vi "Nanonis_SR830_ExternalDevice.vi"(1 "Output Amp #1":dbl=1.0, 2 "Output Amp #2":dbl=1.0, 3 "Output Amp #3":dbl=1.0) -> (7 "X-Value":dbl, 8 "X-Value 2":dbl, 9 "Theta-Value":dbl, 10 "Theta-Value 2":dbl)   [LabVIEW 2021]
uses:
  <instrlib>/Stanford Research 830/Public/Data/Read (All Parameters).vi
  <instrlib>/Stanford Research 830/Stanford Research 830.lvlib
panel:
  in  "External Reference Trigger (0: Sine Zero Crossing)  2":u16(ring) items=["Sine Zero Crossing", "TTL Rising Edge", "TTL Falling Edge"]
  in  "External Reference Trigger (0: Sine Zero Crossing)":u16(ring) items=["Sine Zero Crossing", "TTL Rising Edge", "TTL Falling Edge"]
  in  "External Reference Trigger #2 (0: Sine Zero Crossing)":u16(ring) items=["Sine Zero Crossing", "TTL Rising Edge", "TTL Falling Edge"]
  out "SR830 #3 Sensitivity 3":dbl
  out "SR830 #3 Sensitivity 2":dbl
  out "SR830 #3 Sensitivity":dbl
  out "Sense\nOver 3":bool
  out "Sense\nUnder 3":bool
  out "Sense\nOver 2":bool
  out "Sense\nUnder 2":bool
  out "Sense Under":bool
  out "Sense Over":bool
  in  "Loop Timing (ms)":u32=500
  out "Reference Freq 3":dbl
  out "Theta-Value 3":dbl
  out "R-Value 3":dbl
  out "X-Value 3":dbl
  out "Reference Freq 2":dbl
  out "R-Value 2":dbl
  out "Reference Freq":dbl
  out "R-Value":dbl
  out "Device Intialization":T1
  in  "System #3 Enabled/Disabled":bool
  in  "SR830 #3":refnum<visa-resource-name>="GPIB0::10::INSTR"
  in  "SR830 #3 Input Connection":u16(ring) items=["Single-Ended Voltage", "Differential Voltage", "1 MOhm Current Gain", "100 MOhm Current Gain"]
  in  "SR830 #3\nInput Coupling":u16(ring) items=["AC", "DC"]
  in  "SR830 #3 Input \nShield Grounding":u16(ring) items=["Float", "Ground"]
  in  "SR830 #3 Input\nNotch Filter":u16(ring) items=["None", "Line Notch", "2x Line Notch", "Both Notch Filters"]
  in  "SR830 #3 Trigger Source":u16(ring) items=["Internal", "External"]
  in  "SR830 #3 Internal \nReference Frequency":dbl=17.0
  in  "SR830 #3 Detection Harm. Num.":dbl=1.0
  in  "SR830 #3 Reference Source":u16(ring) items=["External", "Internal"]
  in  "SR830 #3 Manual \nPhase":dbl
  in  "SR830 #3 \nAuto Phase":bool
  in  "SR830 #3 \nTime Constant":u16(ring)=9 items=["10 us", "30 us", "100 us", "300 us", "1 ms", "3 ms", "10 ms", "30 ms", "100 ms", "300 ms", "1 s", "3 s", "10 s", "30 s", "100 s", "300 s", "1 ks", "3 ks", "10 ks", "30 ks"]
  in  "SR830 #3 Low\nPass Filter Slope":u16(ring)=3 items=["6 dB/oct", "12 dB/oct", "18 db/oct", "24 dB/oct"]
  in  "SR830 #3\nSync Filter":bool
  in  "SR830 #3 \nDynamic Reserve":i16(ring)=1 items=["Auto Reserve"=-1, "High Reserve"=0, "Normal"=1, "Low Noise"=2]
  in  "SR830 #3 Initial\nSensitivity":i16(ring)=17 items=["Auto Gain"=-1, "2 nV/fA"=0, "5 nV/fA"=1, "10 nV/fA"=2, "20 nV/fA"=3, "50 nV/fA"=4, "100 nV/fA"=5, "200 nV/fA"=6, "500 nV/fA"=7, "1 uV/pA"=8, "2 uV/pA"=9, "5 uV/pA"=10, "10 uV/pA"=11, "20 uV/pA"=12, "50 uV/pA"=13, "100 uV/pA"=14, "200 uV/pA"=15, "500 uV/pA"=16, "1 mV/nA"=17, "2 mV/nA"=18, "5 mV/nA"=19, "10 mV/nA"=20, "20 mV/nA"=21, "50 mV/nA"=22, "100 mV/nA"=23, "200 mV/nA"=24, "500 mV/mA"=25, "1 V/uA"=26]
  in  "System #2 Enabled/Disabled":bool
  in  "SR830 #2":refnum<visa-resource-name>="GPIB0::10::INSTR"
  in  "SR830 #2 Input Connection":u16(ring)=1 items=["Single-Ended Voltage", "Differential Voltage", "1 MOhm Current Gain", "100 MOhm Current Gain"]
  in  "SR830 #2\nInput Coupling":u16(ring) items=["AC", "DC"]
  in  "SR830 #2 Input \nShield Grounding":u16(ring) items=["Float", "Ground"]
  in  "SR830 #2 Input\nNotch Filter":u16(ring) items=["None", "Line Notch", "2x Line Notch", "Both Notch Filters"]
  in  "SR830 #2 Trigger Source":u16(ring) items=["Internal", "External"]
  in  "SR830 #2 Internal \nReference Frequency":dbl=17.0
  in  "SR830 #2 Detection Harm. Num.":dbl=1.0
  in  "SR830 #2 Reference Source":u16(ring) items=["External", "Internal"]
  in  "SR830 #2 Manual \nPhase":dbl
  in  "SR830 #2 \nAuto Phase":bool
  in  "SR830 #2 \nTime Constant":u16(ring)=8 items=["10 us", "30 us", "100 us", "300 us", "1 ms", "3 ms", "10 ms", "30 ms", "100 ms", "300 ms", "1 s", "3 s", "10 s", "30 s", "100 s", "300 s", "1 ks", "3 ks", "10 ks", "30 ks"]
  in  "SR830 #2 Low\nPass Filter Slope":u16(ring)=3 items=["6 dB/oct", "12 dB/oct", "18 db/oct", "24 dB/oct"]
  in  "SR830 #2\nSync Filter":bool
  in  "SR830 #2 \nDynamic Reserve":i16(ring)=1 items=["Auto Reserve"=-1, "High Reserve"=0, "Normal"=1, "Low Noise"=2]
  in  "SR830 #2 Initial \nSensitivity":i16(ring)=17 items=["Auto Gain"=-1, "2 nV/fA"=0, "5 nV/fA"=1, "10 nV/fA"=2, "20 nV/fA"=3, "50 nV/fA"=4, "100 nV/fA"=5, "200 nV/fA"=6, "500 nV/fA"=7, "1 uV/pA"=8, "2 uV/pA"=9, "5 uV/pA"=10, "10 uV/pA"=11, "20 uV/pA"=12, "50 uV/pA"=13, "100 uV/pA"=14, "200 uV/pA"=15, "500 uV/pA"=16, "1 mV/nA"=17, "2 mV/nA"=18, "5 mV/nA"=19, "10 mV/nA"=20, "20 mV/nA"=21, "50 mV/nA"=22, "100 mV/nA"=23, "200 mV/nA"=24, "500 mV/mA"=25, "1 V/uA"=26]
  in  "SR830 #1 Initial\nSensitivity":i16(ring)=17 items=["Auto Gain"=-1, "2 nV/fA"=0, "5 nV/fA"=1, "10 nV/fA"=2, "20 nV/fA"=3, "50 nV/fA"=4, "100 nV/fA"=5, "200 nV/fA"=6, "500 nV/fA"=7, "1 uV/pA"=8, "2 uV/pA"=9, "5 uV/pA"=10, "10 uV/pA"=11, "20 uV/pA"=12, "50 uV/pA"=13, "100 uV/pA"=14, "200 uV/pA"=15, "500 uV/pA"=16, "1 mV/nA"=17, "2 mV/nA"=18, "5 mV/nA"=19, "10 mV/nA"=20, "20 mV/nA"=21, "50 mV/nA"=22, "100 mV/nA"=23, "200 mV/nA"=24, "500 mV/mA"=25, "1 V/uA"=26]
  in  "SR830 #1 \nDynamic Reserve":i16(ring)=1 items=["Auto Reserve"=-1, "High Reserve"=0, "Normal"=1, "Low Noise"=2]
  in  "SR830 #1\nSync Filter":bool
  in  "SR830 #1 Low\nPass Filter Slope":u16(ring)=3 items=["6 dB/oct", "12 dB/oct", "18 db/oct", "24 dB/oct"]
  in  "SR830 #1 \nTime Constant":u16(ring)=8 items=["10 us", "30 us", "100 us", "300 us", "1 ms", "3 ms", "10 ms", "30 ms", "100 ms", "300 ms", "1 s", "3 s", "10 s", "30 s", "100 s", "300 s", "1 ks", "3 ks", "10 ks", "30 ks"]
  in  "SR830 #1 \nAuto Phase":bool
  in  "SR830 #1 Manual \nPhase":dbl
  in  "SR830 #1 Reference Source":u16(ring)=1 items=["External", "Internal"]
  in  "SR830 #1 Detection Harm. Num.":dbl=1.0
  in  "SR830 #1 Internal \nReference Frequency":dbl=17.0
  in  "SR830 #1 Trigger Source":u16(ring) items=["Internal", "External"]
  in  "SR830 #1 Input\nNotch Filter":u16(ring) items=["None", "Line Notch", "2x Line Notch", "Both Notch Filters"]
  in  "SR830 #1 Input \nShield Grounding":u16(ring) items=["Float", "Ground"]
  in  "SR830 #1\nInput Coupling":u16(ring) items=["AC", "DC"]
  in  "SR830 #1 Input Connection":u16(ring)=1 items=["Single-Ended Voltage", "Differential Voltage", "1 MOhm Current Gain", "100 MOhm Current Gain"]
  in  "SR830 #1":refnum<visa-resource-name>="GPIB0::10::INSTR"
  in  "System #1 Enabled/Disabled":bool
  in  "System Reset All?":bool
  in  "program_stop":bool
  # "Readout (Recorded)"
  # "SR830"
  # "SR830"
  # "SR830"
  # "Input Signal"
  # "Input Signal"
  # "Input Signal"
  # "Readout (Recorded)"
  # "Readout (Recorded)"
  # "Source / Reference"
  # "Source / Reference"
  # "Source / Reference"
  # "Input Filters & Sens"
  # "Input Filters & Sens"
  # "Input Filters & Sens"
  # "Initialisation:\n--> Reset \n--> Instruments?"
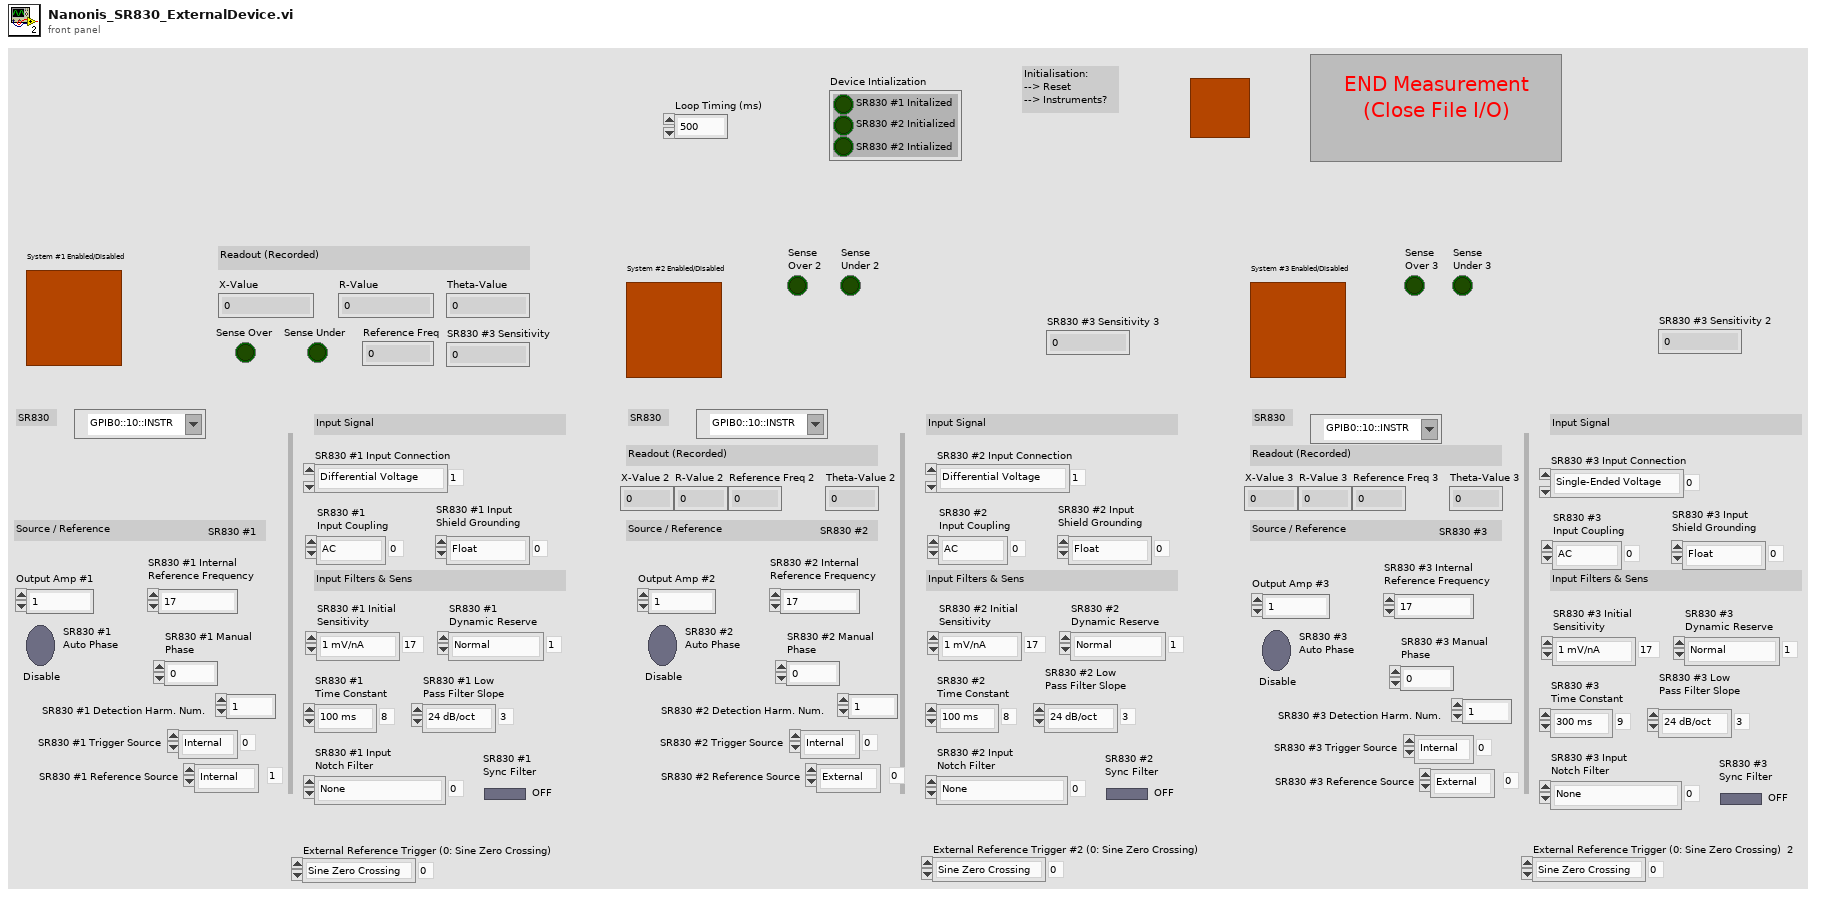
[diagram p1: front panel]
types:
  T1 = cluster{"SR830 #1 Initalized":bool, "SR830 #2 Initialized":bool, "SR830 #2 Intialized":bool}
  T2 = cluster{"VISA resource name out":refnum<visa-resource-name>, "error out":errorcluster}
  T3 = cluster{"Initialised?":bool, "Initialised?":bool, "Initialised?":bool}
  T4 = cluster{"Reference & Errors":cluster{"VISA resource name out":refnum<visa-resource-name>, "error out":errorcluster}, "Reference & Errors":cluster{"VISA resource name out":refnum<visa-resource-name>, "error out":errorcluster}, "Reference & Errors":cluster{"VISA resource name out":refnum<visa-resource-name>, "error out":errorcluster}}
  T5 = cluster{"Voltage Output":dbl, "Voltage Output":dbl, "Voltage Output":dbl}
  T6 = cluster{"Sensitivity":i16, "Sensitivity":i16, "Sensitivity":i16}
  T7 = cluster{"System #1 Enabled/Disabled":bool, "System #2 Enabled/Disabled":bool, "System #3 Enabled/Disabled":bool}
  T8 = cluster{"X-Value":dbl, "Y-Value":dbl, "R-Value":dbl, "Theta-Value":dbl, "Aux In 1 Value":dbl, "Aux In 2 Value":dbl, "Aux In 3 Value":dbl, "Aux In 4 Value":dbl, "Reference Frequency":dbl, "Channel 1 Display":dbl, "Channel 2 Display":dbl}
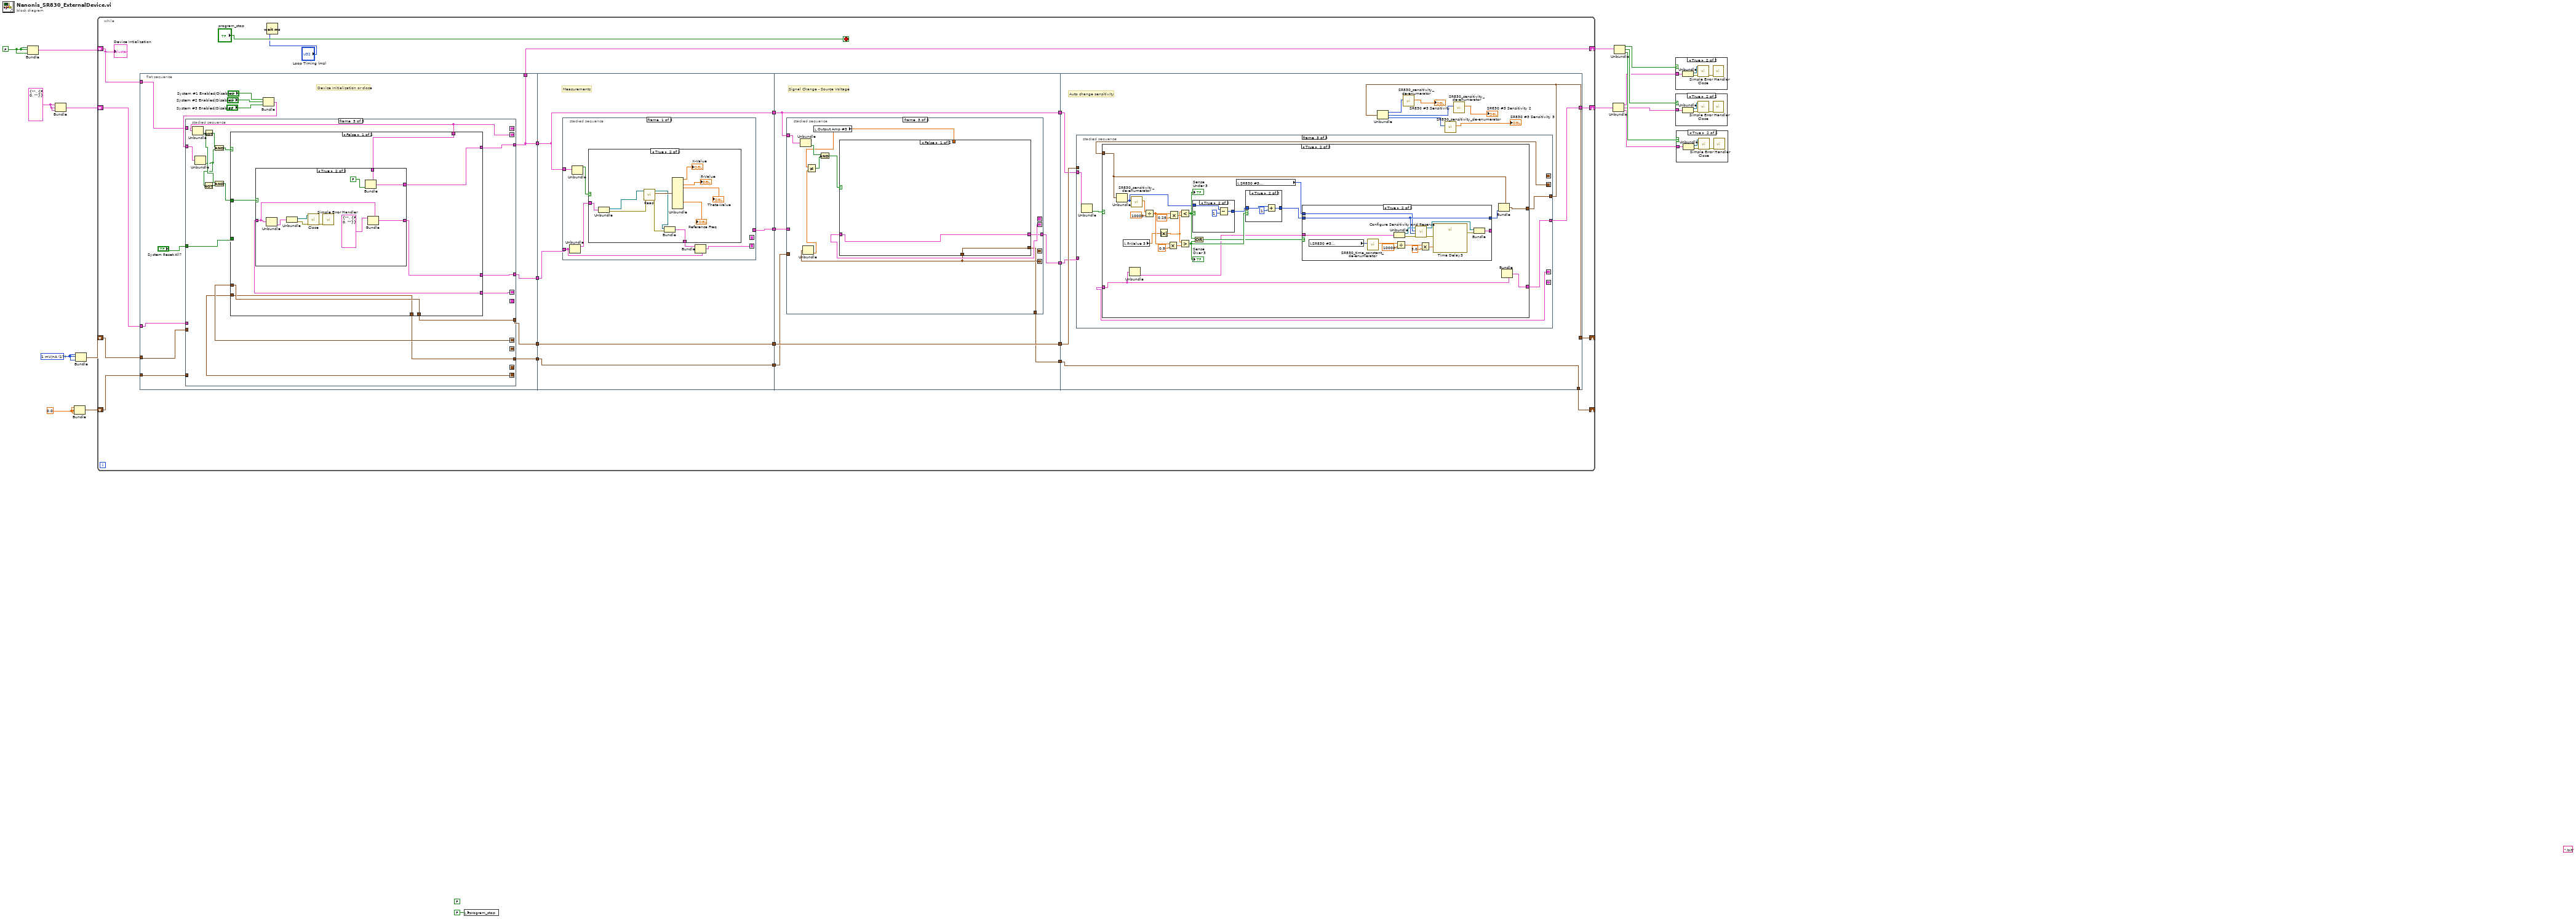
[diagram p0: block diagram]
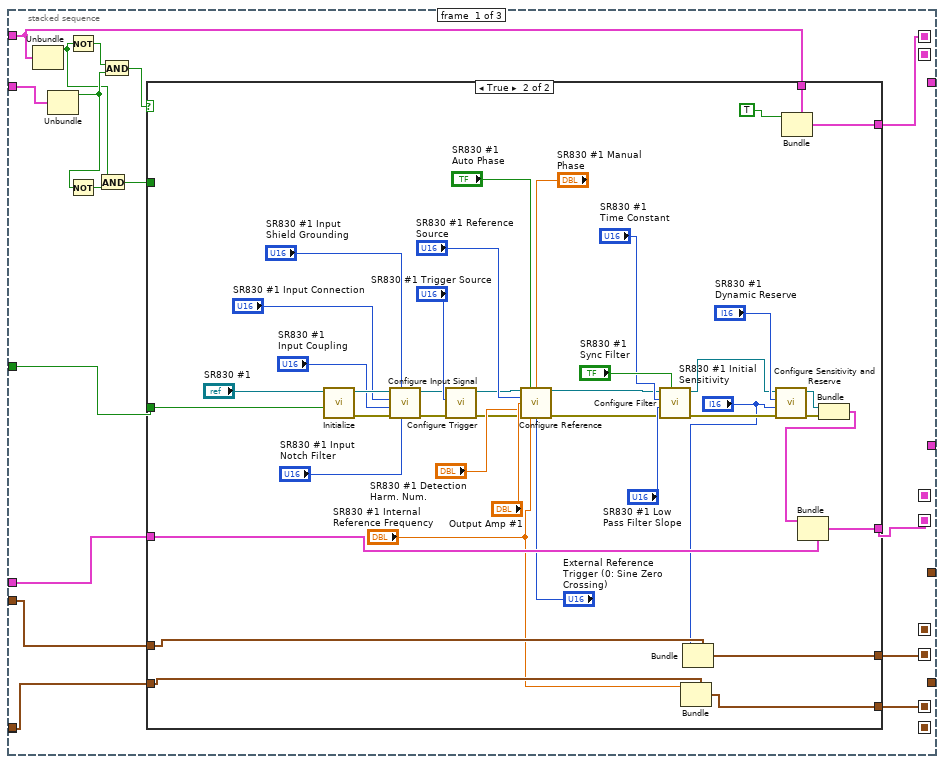
[diagram p5: hidden frame]
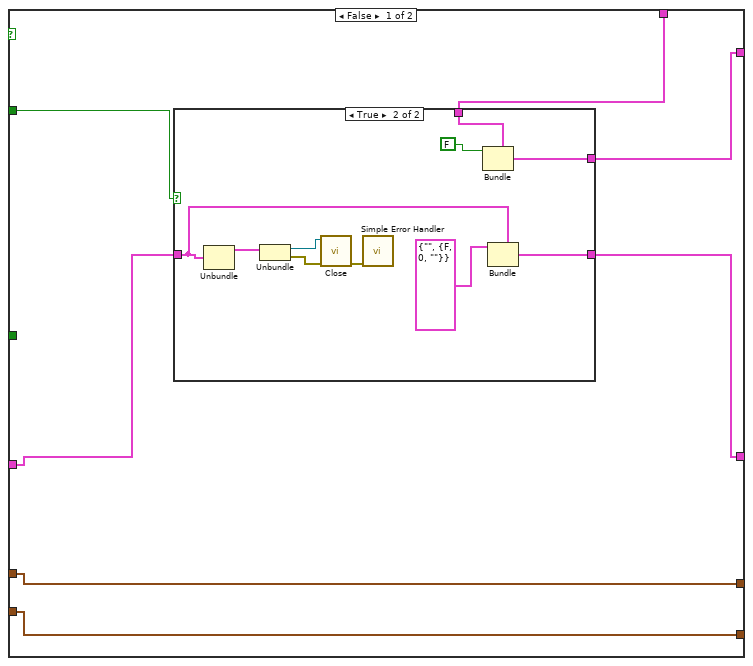
[diagram p6: hidden frame]
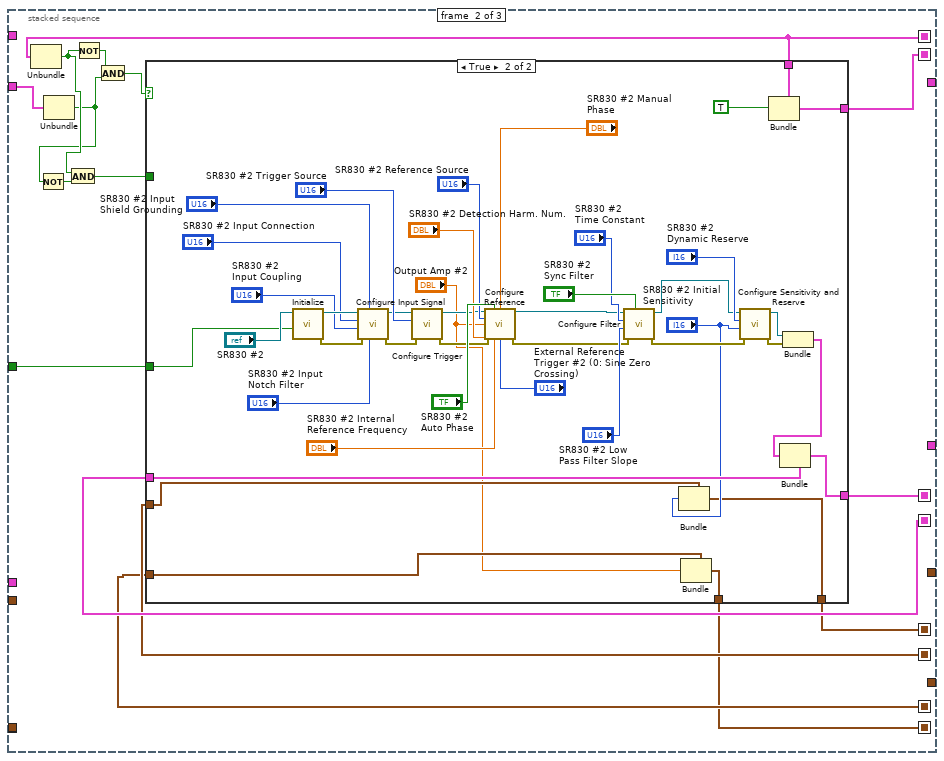
[diagram p8: hidden frame]
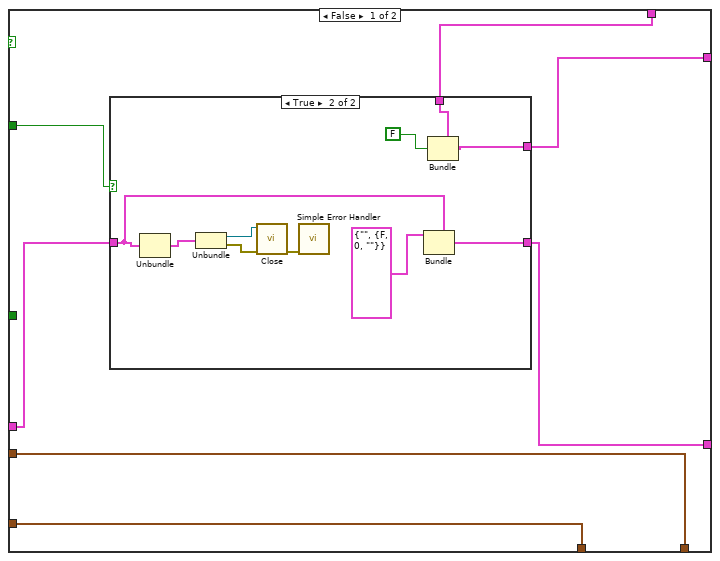
[diagram p9: hidden frame]
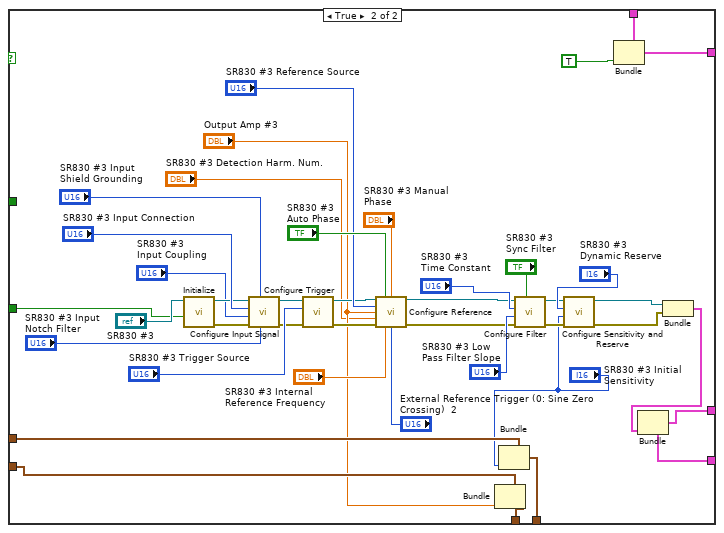
[diagram p12: hidden frame]
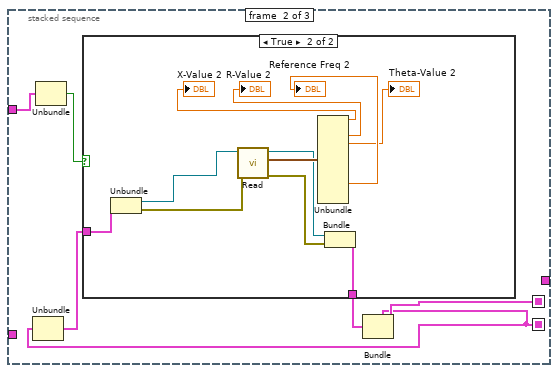
[diagram p14: hidden frame]
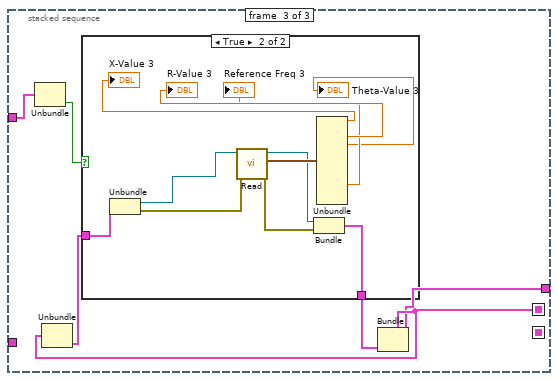
[diagram p16: hidden frame]
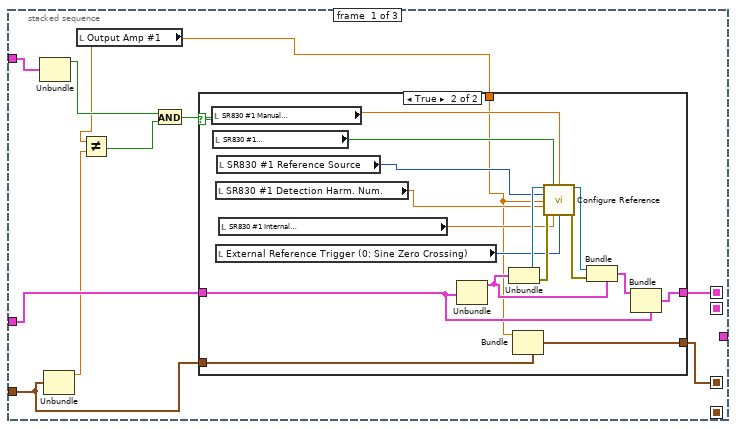
[diagram p18: hidden frame]
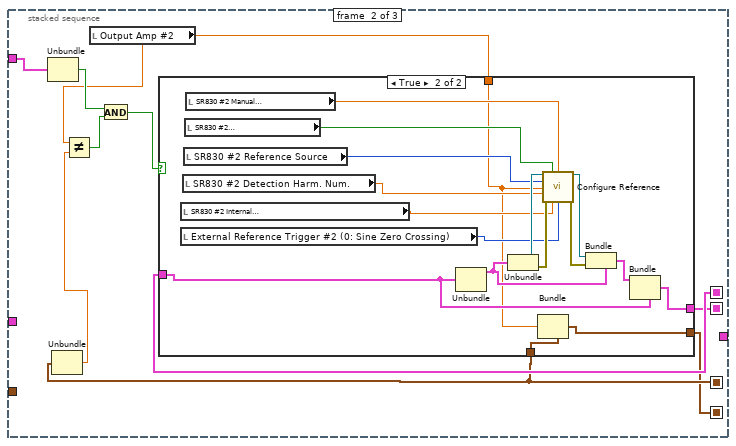
[diagram p20: hidden frame]
diagram:
  w2 = 0.0 ("Voltage Output")
  w4 = i16 17 items=["Auto Gain"=-1, "2 nV/fA"=0, "5 nV/fA"=1, "10 nV/fA"=2, "20 nV/fA"=3, "50 nV/fA"=4, "100 nV/fA"=5, "200 nV/fA"=6, "500 nV/fA"=7, "1 uV/pA"=8, "2 uV/pA"=9, "5 uV/pA"=10, "10 uV/pA"=11, "20 uV/pA"=12, "50 uV/pA"=13, "100 uV/pA"=14, "200 uV/pA"=15, "500 uV/pA"=16, "1 mV/nA"=17, "2 mV/nA"=18, "5 mV/nA"=19, "10 mV/nA"=20, "20 mV/nA"=21, "50 mV/nA"=22, "100 mV/nA"=23, "200 mV/nA"=24, "500 mV/mA"=25, "1 V/uA"=26] ("Sensitivity")
  w14 = T2 {"VISA resource name out"="", "error out"={"status"=FALSE, "code"=0, "source"=""}} ("Reference & Errors")
  w16 = FALSE ("Initialised?")
  (unwired) ".txt"
  (unwired) FALSE ("Measuring")
  n1 = Bundle("Initialised?"=w16, "Initialised?"=w16, "Initialised?"=w16) -> (w15:T3)  [unwired: 1 in]
  n2 = Bundle("Reference & Errors"=w14, "Reference & Errors"=w14, "Reference & Errors"=w14) -> (w13:T4)  [unwired: 1 in]
  n3 = Bundle("Voltage Output"=w2, "Voltage Output"=w2, "Voltage Output"=w2) -> (w1:T5)  [unwired: 1 in]
  n4 = Bundle("Sensitivity"=w4, "Sensitivity"=w4, "Sensitivity"=w4) -> (w3:T6)  [unwired: 1 in]
  n5 = while {
    shift-right: [w34] -> w12
    shift-left: w15 -> [w38]
    shift-right: [w18] -> w11
    shift-left: w13 -> [w37]
    shift-right: [w30] -> _
    shift-left: w3 -> [w32]
    shift-right: [w19] -> _
    shift-left: w1 -> [w24]
    stop <- "program_stop" stop-if-true
    n6 = flat-sequence {
      tunnel: w38 -> [w47]
      tunnel: w37 -> [w46]
      tunnel: [w44] -> w36
      tunnel: [w45] -> w35
      tunnel: [w45] -> w34
      tunnel: w32 -> [w43]
      tunnel: [w42] -> w31
      tunnel: w24 -> [w41]
      tunnel: [w40] -> w23
      tunnel: w36 -> [w285]
      tunnel: w35 -> [w282]
      tunnel: [w284] -> w29
      tunnel: w31 -> [w283]
      tunnel: [w283] -> w28
      tunnel: [w282] -> w26
      tunnel: w23 -> [w281]
      tunnel: [w281] -> w22
      tunnel: w29 -> [w342]
      tunnel: w28 -> [w345]
      tunnel: [w345] -> w27
      tunnel: w26 -> [w343]
      tunnel: [w343] -> w25
      tunnel: w22 -> [w344]
      tunnel: [w341] -> w21
      tunnel: [w340] -> w20
      tunnel: w27 -> [w444]
      tunnel: [w443] -> w30
      tunnel: [w442] -> w18
      tunnel: w25 -> [w441]
      tunnel: w21 -> [w434]
      tunnel: w20 -> [w433]
      tunnel: [w433] -> w19
      frame #0 {
        # "Device Initialization or close"
        n7 = Bundle("System #1 Enabled/Disabled"="System #1 Enabled/Disabled", "System #2 Enabled/Disabled"="System #2 Enabled/Disabled", "System #3 Enabled/Disabled"="System #3 Enabled/Disabled") -> (w48:T7)  [unwired: 1 in]
        n8 = stacked-sequence {
          seq-local: [w63 _ _] -> [_ w140 _]
          seq-local: [_ w139 _] -> [_ _ w216]
          seq-local: [w62 _ _] -> [_ w138 _]
          seq-local: [_ w137 _] -> [_ _ w214]
          seq-local: [w55 _ _] -> [_ w132 _]
          seq-local: [_ w131 _] -> [_ _ w208]
          seq-local: [_ w129 _] -> [_ _ w206]
          seq-local: [w53 _ _] -> [_ w130 _]
          tunnel: "System Reset All?" -> [w68 w144 w220]
          tunnel: w48 -> [w67 w143 w218]
          tunnel: w47 -> [w64 _ _]
          tunnel: w46 -> [w57 _ _]
          tunnel: [_ _ w215] -> w45
          tunnel: [_ _ w213] -> w44
          tunnel: w43 -> [w56 _ _]
          tunnel: [_ _ w207] -> w42
          tunnel: [w54 _ _] -> _
          tunnel: w41 -> [w54 _ _]
          tunnel: [_ _ w205] -> w40
          frame #0 {
            n9 = Unbundle(w64) -> ("Initialised?"=w59:bool)  [unwired: 2 out]
            n10 = Unbundle(w67) -> ("System #1 Enabled/Disabled"=w60:bool)  [unwired: 2 out]
            n11 = Not(x=w59) -> (.not. x?=w66:bool)
            n12 = Not(x=w60) -> (.not. x?=w61:bool)
            n13 = And(x=w59, y=w61) -> (x .and. y?=w58:bool)
            n14 = And(x=w66, y=w60) -> (x .and. y?=w65:bool)
            n15 = case shown="True" w65 {
              tunnel: w68 -> [_ w101]
              tunnel: w64 -> [w73 w100]
              tunnel: [w72 w99] -> w63
              tunnel: w57 -> [w75 w97]
              tunnel: [w74 w95] -> w62
              tunnel: w58 -> [w71 _]
              tunnel: w56 -> [w70 w94]
              tunnel: [w70 w93] -> w55
              tunnel: w54 -> [w69 w91]
              tunnel: [w69 w90] -> w53
              frame False {
                n16 = case shown="True" w71 {
                  tunnel: w75 -> [w77 w84]
                  tunnel: [w77 w82] -> w74
                  tunnel: w73 -> [w76 w79]
                  tunnel: [w76 w78] -> w72
                  frame False {
                  }
                  frame True {
                    n17 = Unbundle(w84) -> ("Reference & Errors"=w81:T2)  [unwired: 2 out]
                    n18 = Unbundle(w81) -> ("VISA resource name out"=w86:refnum<visa-resource-name>, "error out"=w85:errorcluster)
                    n19 = call <instrlib>:"Close.vi"("error in (no error)"=w85, "VISA resource name"=w86) -> ("error out"=w87:errorcluster)  [unwired: 9 in]
                    n20 = call <vilib>:"Simple Error Handler.vi"("error in (no error)"=w87) -> ()  [unwired: 4 in, 5 out]
                    n21 = Bundle(cluster=w79, "Initialised?"=FALSE) -> (w78:T3)  [unwired: 2 in]
                    n22 = Bundle(cluster=w84, "Reference & Errors"=T2 {"VISA resource name out"="", "error out"={"status"=FALSE, "code"=0, "source"=""}}) -> (w82:T4)  [unwired: 2 in]
                  }
                }
              }
              frame True {
                n23 = call <instrlib>:"Initialize.vi"("Reset (True)"=w101, "VISA resource name"="SR830 #1") -> ("error out"=w106:errorcluster, "VISA resource name out"=w105:refnum<visa-resource-name>)  [unwired: 8 in]
                n24 = call <instrlib>:"Configure Input Signal.vi"("Input Notch Filter (0: None)"="SR830 #1 Input\nNotch Filter", "Input Shield Grounding (0: Float)"="SR830 #1 Input \nShield Grounding", "error in (no error)"=w106, "Input Coupling (0: AC)"="SR830 #1\nInput Coupling", "Input Connection (0: Single-Ended Voltage)"="SR830 #1 Input Connection", "VISA resource name"=w105) -> ("error out"=w108:errorcluster, "VISA resource name out"=w107:refnum<visa-resource-name>)  [unwired: 4 in]
                n25 = call <instrlib>:"Configure Trigger.vi"("error in (no error)"=w108, "Trigger Source (0: Internal)"="SR830 #1 Trigger Source", "VISA resource name"=w107) -> ("error out"=w110:errorcluster, "VISA resource name out"=w109:refnum<visa-resource-name>)  [unwired: 7 in]
                n26 = call <instrlib>:"Configure Reference.vi"("VISA resource name"=w109, "Auto Phase (T: Enabled)"="SR830 #1 \nAuto Phase", "Manual Phase (0 Degree)"="SR830 #1 Manual \nPhase", "Reference Source (1: Internal)"="SR830 #1 Reference Source", "Sine Output Amplitude (1 V)"="Output Amp #1", "Detection Harmonic Number (1)"="SR830 #1 Detection Harm. Num.", "error in (no error)"=w110, "Internal Reference Frequency (1000 Hz)"="SR830 #1 Internal \nReference Frequency", "External Reference Trigger (0: Sine Zero Crossing)"="External Reference Trigger (0: Sine Zero Crossing)") -> ("VISA resource name out"=w112:refnum<visa-resource-name>, "error out"=w111:errorcluster)  [unwired: 5 in]
                n27 = call <instrlib>:"Configure Filter.vi"("Enable Sync Filter (F: Disable)"="SR830 #1\nSync Filter", "error in (no error)"=w111, "Low Pass Filter Slope (1: 12dB/oct)"="SR830 #1 Low\nPass Filter Slope", "Time Constant (8: 100ms)"="SR830 #1 \nTime Constant", "VISA resource name"=w112) -> ("error out"=w125:errorcluster, "VISA resource name out"=w124:refnum<visa-resource-name>)  [unwired: 5 in]
                n28 = Bundle(cluster=w91, "Voltage Output"="SR830 #1 Internal \nReference Frequency") -> (w90:T5)  [unwired: 2 in]
                n29 = Bundle(cluster=w94, "Sensitivity"="SR830 #1 Initial\nSensitivity") -> (w93:T6)  [unwired: 2 in]
                n30 = call <instrlib>:"Configure Sensitivity and Reserve.vi"("error in (no error)"=w125, "Sensitivity (-1: Auto gain)"="SR830 #1 Initial\nSensitivity", "Dynamic Reserve (-1: Auto Reserve)"="SR830 #1 \nDynamic Reserve", "VISA resource name"=w124) -> ("error out"=w128:errorcluster, "VISA resource name out"=w127:refnum<visa-resource-name>)  [unwired: 6 in]
                n31 = Bundle(cluster=w100, "Initialised?"=TRUE) -> (w99:T3)  [unwired: 2 in]
                n32 = Bundle("VISA resource name out"=w127, "error out"=w128) -> (w96:T2)  [unwired: 1 in]
                n33 = Bundle(cluster=w97, "Reference & Errors"=w96) -> (w95:T4)  [unwired: 2 in]
              }
            }
          }
          frame #1 {
            n34 = Unbundle(w140) -> ("Initialised?"=w134:bool)  [unwired: 2 out]
            n35 = Unbundle(w143) -> ("System #2 Enabled/Disabled"=w133:bool)  [unwired: 2 out]
            n36 = Not(x=w133) -> (.not. x?=w136:bool)
            n37 = And(x=w134, y=w136) -> (x .and. y?=w135:bool)
            n38 = Not(x=w134) -> (.not. x?=w142:bool)
            n39 = And(x=w142, y=w133) -> (x .and. y?=w141:bool)
            n40 = case shown="True" w141 {
              tunnel: w144 -> [_ w177]
              tunnel: w140 -> [w149 w176]
              tunnel: [w148 w174] -> w139
              tunnel: w138 -> [w151 w172]
              tunnel: [w150 w171] -> w137
              tunnel: w135 -> [w147 _]
              tunnel: w132 -> [w146 w170]
              tunnel: [w146 w168] -> w131
              tunnel: w130 -> [w145 w167]
              tunnel: [w145 w165] -> w129
              frame False {
                n41 = case shown="True" w147 {
                  tunnel: w151 -> [w153 w160]
                  tunnel: [w153 w158] -> w150
                  tunnel: w149 -> [w152 w156]
                  tunnel: [w152 w155] -> w148
                  frame False {
                  }
                  frame True {
                    n42 = Unbundle(w160) -> ("Reference & Errors"=w157:T2)  [unwired: 2 out]
                    n43 = Unbundle(w157) -> ("VISA resource name out"=w162:refnum<visa-resource-name>, "error out"=w161:errorcluster)
                    n44 = call <instrlib>:"Close.vi"("error in (no error)"=w161, "VISA resource name"=w162) -> ("error out"=w163:errorcluster)  [unwired: 9 in]
                    n45 = call <vilib>:"Simple Error Handler.vi"("error in (no error)"=w163) -> ()  [unwired: 4 in, 5 out]
                    n46 = Bundle(cluster=w160, "Reference & Errors"=T2 {"VISA resource name out"="", "error out"={"status"=FALSE, "code"=0, "source"=""}}) -> (w158:T4)  [unwired: 2 in]
                    n47 = Bundle(cluster=w156, "Initialised?"=FALSE) -> (w155:T3)  [unwired: 2 in]
                  }
                }
              }
              frame True {
                n48 = call <instrlib>:"Initialize.vi"("Reset (True)"=w177, "VISA resource name"="SR830 #2") -> ("error out"=w182:errorcluster, "VISA resource name out"=w181:refnum<visa-resource-name>)  [unwired: 8 in]
                n49 = call <instrlib>:"Configure Input Signal.vi"("Input Notch Filter (0: None)"="SR830 #2 Input\nNotch Filter", "Input Shield Grounding (0: Float)"="SR830 #2 Input \nShield Grounding", "error in (no error)"=w182, "Input Coupling (0: AC)"="SR830 #2\nInput Coupling", "Input Connection (0: Single-Ended Voltage)"="SR830 #2 Input Connection", "VISA resource name"=w181) -> ("error out"=w184:errorcluster, "VISA resource name out"=w183:refnum<visa-resource-name>)  [unwired: 4 in]
                n50 = call <instrlib>:"Configure Trigger.vi"("error in (no error)"=w184, "Trigger Source (0: Internal)"="SR830 #2 Trigger Source", "VISA resource name"=w183) -> ("error out"=w186:errorcluster, "VISA resource name out"=w185:refnum<visa-resource-name>)  [unwired: 7 in]
                n51 = call <instrlib>:"Configure Reference.vi"("VISA resource name"=w185, "Auto Phase (T: Enabled)"="SR830 #2 \nAuto Phase", "Manual Phase (0 Degree)"="SR830 #2 Manual \nPhase", "Reference Source (1: Internal)"="SR830 #2 Reference Source", "Sine Output Amplitude (1 V)"="Output Amp #2", "Detection Harmonic Number (1)"="SR830 #2 Detection Harm. Num.", "error in (no error)"=w186, "Internal Reference Frequency (1000 Hz)"="SR830 #2 Internal \nReference Frequency", "External Reference Trigger (0: Sine Zero Crossing)"="External Reference Trigger #2 (0: Sine Zero Crossing)") -> ("VISA resource name out"=w188:refnum<visa-resource-name>, "error out"=w187:errorcluster)  [unwired: 5 in]
                n52 = call <instrlib>:"Configure Filter.vi"("Enable Sync Filter (F: Disable)"="SR830 #2\nSync Filter", "error in (no error)"=w187, "Low Pass Filter Slope (1: 12dB/oct)"="SR830 #2 Low\nPass Filter Slope", "Time Constant (8: 100ms)"="SR830 #2 \nTime Constant", "VISA resource name"=w188) -> ("error out"=w201:errorcluster, "VISA resource name out"=w200:refnum<visa-resource-name>)  [unwired: 5 in]
                n53 = Bundle(cluster=w170, "Sensitivity"="SR830 #2 Initial \nSensitivity") -> (w168:T6)  [unwired: 2 in]
                n54 = Bundle(cluster=w167, "Voltage Output"="Output Amp #2") -> (w165:T5)  [unwired: 2 in]
                n55 = call <instrlib>:"Configure Sensitivity and Reserve.vi"("error in (no error)"=w201, "Sensitivity (-1: Auto gain)"="SR830 #2 Initial \nSensitivity", "Dynamic Reserve (-1: Auto Reserve)"="SR830 #2 \nDynamic Reserve", "VISA resource name"=w200) -> ("error out"=w204:errorcluster, "VISA resource name out"=w203:refnum<visa-resource-name>)  [unwired: 6 in]
                n56 = Bundle(cluster=w176, "Initialised?"=TRUE) -> (w174:T3)  [unwired: 2 in]
                n57 = Bundle("VISA resource name out"=w203, "error out"=w204) -> (w173:T2)  [unwired: 1 in]
                n58 = Bundle(cluster=w172, "Reference & Errors"=w173) -> (w171:T4)  [unwired: 2 in]
              }
            }
          }
          frame #2 {
            n59 = Unbundle(w216) -> ("Initialised?"=w211:bool)  [unwired: 2 out]
            n60 = Unbundle(w218) -> ("System #3 Enabled/Disabled"=w210:bool)  [unwired: 2 out]
            n61 = Not(x=w210) -> (.not. x?=w212:bool)
            n62 = Not(x=w211) -> (.not. x?=w219:bool)
            n63 = And(x=w219, y=w210) -> (x .and. y?=w217:bool)
            n64 = And(x=w211, y=w212) -> (x .and. y?=w209:bool)
            n65 = case shown="False" w217 {
              tunnel: w220 -> [_ w254]
              tunnel: w216 -> [w224 w253]
              tunnel: [w223 w252] -> w215
              tunnel: w209 -> [w227 _]
              tunnel: w214 -> [w226 w250]
              tunnel: [w225 w249] -> w213
              tunnel: w208 -> [w222 w247]
              tunnel: [w222 w246] -> w207
              tunnel: w206 -> [w221 w244]
              tunnel: [w221 w242] -> w205
              frame False {
                n66 = case shown="True" w227 {
                  tunnel: w226 -> [w229 w236]
                  tunnel: [w229 w234] -> w225
                  tunnel: w224 -> [w228 w232]
                  tunnel: [w228 w231] -> w223
                  frame False {
                  }
                  frame True {
                    n67 = Unbundle(w236) -> ("Reference & Errors"=w233:T2)  [unwired: 2 out]
                    n68 = Unbundle(w233) -> ("VISA resource name out"=w238:refnum<visa-resource-name>, "error out"=w237:errorcluster)
                    n69 = call <instrlib>:"Close.vi"("error in (no error)"=w237, "VISA resource name"=w238) -> ("error out"=w239:errorcluster)  [unwired: 9 in]
                    n70 = call <vilib>:"Simple Error Handler.vi"("error in (no error)"=w239) -> ()  [unwired: 4 in, 5 out]
                    n71 = Bundle(cluster=w232, "Initialised?"=FALSE) -> (w231:T3)  [unwired: 2 in]
                    n72 = Bundle(cluster=w236, "Reference & Errors"=T2 {"VISA resource name out"="", "error out"={"status"=FALSE, "code"=0, "source"=""}}) -> (w234:T4)  [unwired: 2 in]
                  }
                }
              }
              frame True {
                n73 = call <instrlib>:"Initialize.vi"("Reset (True)"=w254, "VISA resource name"="SR830 #3") -> ("error out"=w258:errorcluster, "VISA resource name out"=w257:refnum<visa-resource-name>)  [unwired: 8 in]
                n74 = call <instrlib>:"Configure Input Signal.vi"("Input Notch Filter (0: None)"="SR830 #3 Input\nNotch Filter", "Input Shield Grounding (0: Float)"="SR830 #3 Input \nShield Grounding", "error in (no error)"=w258, "Input Coupling (0: AC)"="SR830 #3\nInput Coupling", "Input Connection (0: Single-Ended Voltage)"="SR830 #3 Input Connection", "VISA resource name"=w257) -> ("error out"=w260:errorcluster, "VISA resource name out"=w259:refnum<visa-resource-name>)  [unwired: 4 in]
                n75 = call <instrlib>:"Configure Trigger.vi"("error in (no error)"=w260, "Trigger Source (0: Internal)"="SR830 #3 Trigger Source", "VISA resource name"=w259) -> ("error out"=w262:errorcluster, "VISA resource name out"=w261:refnum<visa-resource-name>)  [unwired: 7 in]
                n76 = call <instrlib>:"Configure Reference.vi"("VISA resource name"=w261, "Auto Phase (T: Enabled)"="SR830 #3 \nAuto Phase", "Manual Phase (0 Degree)"="SR830 #3 Manual \nPhase", "Reference Source (1: Internal)"="SR830 #3 Reference Source", "Sine Output Amplitude (1 V)"="Output Amp #3", "Detection Harmonic Number (1)"="SR830 #3 Detection Harm. Num.", "error in (no error)"=w262, "Internal Reference Frequency (1000 Hz)"="SR830 #3 Internal \nReference Frequency", "External Reference Trigger (0: Sine Zero Crossing)"="External Reference Trigger (0: Sine Zero Crossing)  2") -> ("VISA resource name out"=w264:refnum<visa-resource-name>, "error out"=w263:errorcluster)  [unwired: 5 in]
                n77 = Bundle(cluster=w244, "Voltage Output"="Output Amp #3") -> (w242:T5)  [unwired: 2 in]
                n78 = Bundle(cluster=w247, "Sensitivity"="SR830 #3 Initial\nSensitivity") -> (w246:T6)  [unwired: 2 in]
                n79 = call <instrlib>:"Configure Filter.vi"("Enable Sync Filter (F: Disable)"="SR830 #3\nSync Filter", "error in (no error)"=w263, "Low Pass Filter Slope (1: 12dB/oct)"="SR830 #3 Low\nPass Filter Slope", "Time Constant (8: 100ms)"="SR830 #3 \nTime Constant", "VISA resource name"=w264) -> ("error out"=w276:errorcluster, "VISA resource name out"=w275:refnum<visa-resource-name>)  [unwired: 5 in]
                n80 = call <instrlib>:"Configure Sensitivity and Reserve.vi"("error in (no error)"=w276, "Sensitivity (-1: Auto gain)"="SR830 #3 Initial\nSensitivity", "Dynamic Reserve (-1: Auto Reserve)"="SR830 #3 \nDynamic Reserve", "VISA resource name"=w275) -> ("error out"=w278:errorcluster, "VISA resource name out"=w277:refnum<visa-resource-name>)  [unwired: 6 in]
                n81 = Bundle(cluster=w253, "Initialised?"=TRUE) -> (w252:T3)  [unwired: 2 in]
                n82 = Bundle("VISA resource name out"=w277, "error out"=w278) -> (w248:T2)  [unwired: 1 in]
                n83 = Bundle(cluster=w250, "Reference & Errors"=w248) -> (w249:T4)  [unwired: 2 in]
              }
            }
          }
        }
      }
      frame #1 {
        # "Measurements"
        n84 = stacked-sequence {
          seq-local: [_ w307 _] -> [_ _ w325]
          seq-local: [w289 _ _] -> [_ w305 _]
          tunnel: w282 -> [w288 w308 w327]
          tunnel: w285 -> [w290 _ _]
          tunnel: [_ _ w322] -> w284
          frame #0 {
            n85 = Unbundle(w290) -> ("Reference & Errors"=w286:T2)  [unwired: 2 out]
            n86 = Unbundle(w288) -> ("Initialised?"=w291:bool)  [unwired: 2 out]
            n87 = case shown="True" w291 {
              tunnel: [w292 w298] -> w287
              tunnel: w286 -> [w292 w297]
              frame False {
              }
              frame True {
                n88 = Unbundle(w297) -> ("VISA resource name out"=w303:refnum<visa-resource-name>, "error out"=w302:errorcluster)
                n89 = call-poly <instrlib>:"Read.vi"("error in (no error)"=w302, "VISA resource name"=w303) -> ("error out"=w300:errorcluster, "Parameter Values"=w301:T8, "VISA resource name out"=w299:refnum<visa-resource-name>)  [unwired: 7 in]
                n90 = Bundle("VISA resource name out"=w299, "error out"=w300) -> (w298:T2)  [unwired: 1 in]
                n91 = Unbundle(w301) -> ("X-Value"=→"X-Value":dbl, "R-Value"=→"R-Value":dbl, "Theta-Value"=→"Theta-Value":dbl, "Reference Frequency"=→"Reference Freq":dbl)  [unwired: 7 out]
              }
            }
            n92 = Bundle(cluster=w290, "Reference & Errors"=w287) -> (w289:T4)  [unwired: 2 in]
          }
          frame #1 {
            n93 = Unbundle(w305) -> ("Reference & Errors"=w306:T2)  [unwired: 2 out]
            n94 = Unbundle(w308) -> ("Initialised?"=w309:bool)  [unwired: 2 out]
            n95 = case shown="True" w309 {
              tunnel: w306 -> [w310 w321]
              tunnel: [w310 w315] -> w304
              frame False {
              }
              frame True {
                n96 = Unbundle(w321) -> ("VISA resource name out"=w320:refnum<visa-resource-name>, "error out"=w319:errorcluster)
                n97 = call-poly <instrlib>:"Read.vi"("error in (no error)"=w319, "VISA resource name"=w320) -> ("error out"=w316:errorcluster, "Parameter Values"=w318:T8, "VISA resource name out"=w317:refnum<visa-resource-name>)  [unwired: 7 in]
                n98 = Unbundle(w318) -> ("X-Value"=→"X-Value 2":dbl, "R-Value"=→"R-Value 2":dbl, "Theta-Value"=→"Theta-Value 2":dbl, "Reference Frequency"=→"Reference Freq 2":dbl)  [unwired: 7 out]
                n99 = Bundle("VISA resource name out"=w317, "error out"=w316) -> (w315:T2)  [unwired: 1 in]
              }
            }
            n100 = Bundle(cluster=w305, "Reference & Errors"=w304) -> (w307:T4)  [unwired: 2 in]
          }
          frame #2 {
            n101 = Unbundle(w327) -> ("Initialised?"=w326:bool)  [unwired: 2 out]
            n102 = Unbundle(w325) -> ("Reference & Errors"=w324:T2)  [unwired: 2 out]
            n103 = case shown="True" w326 {
              tunnel: w324 -> [w328 w339]
              tunnel: [w328 w333] -> w323
              frame False {
              }
              frame True {
                n104 = Unbundle(w339) -> ("VISA resource name out"=w338:refnum<visa-resource-name>, "error out"=w337:errorcluster)
                n105 = call-poly <instrlib>:"Read.vi"("error in (no error)"=w337, "VISA resource name"=w338) -> ("error out"=w334:errorcluster, "Parameter Values"=w336:T8, "VISA resource name out"=w335:refnum<visa-resource-name>)  [unwired: 7 in]
                n106 = Bundle("VISA resource name out"=w335, "error out"=w334) -> (w333:T2)  [unwired: 1 in]
                n107 = Unbundle(w336) -> ("X-Value"=→"X-Value 3":dbl, "R-Value"=→"R-Value 3":dbl, "Theta-Value"=→"Theta-Value 3":dbl, "Reference Frequency"=→"Reference Freq 3":dbl)  [unwired: 7 out]
              }
            }
            n108 = Bundle(cluster=w325, "Reference & Errors"=w323) -> (w322:T4)  [unwired: 2 in]
          }
        }
      }
      frame #2 {
        # "Signal Change - Source Voltage"
        n109 = stacked-sequence {
          seq-local: [w352 _ _] -> [_ w382 _]
          seq-local: [_ w378 _] -> [_ _ w408]
          seq-local: [w346 _ _] -> [_ w376 _]
          seq-local: [_ w375 _] -> [_ _ w405]
          tunnel: w344 -> [w347 _ _]
          tunnel: w343 -> [w351 w381 w411]
          tunnel: w342 -> [w353 _ _]
          tunnel: [_ _ w407] -> w341
          tunnel: [_ _ w404] -> w340
          frame #0 {
            n110 = Unbundle(w351) -> ("Initialised?"=w350:bool)  [unwired: 2 out]
            n111 = Unbundle(w347) -> ("Voltage Output"=w349:dbl)  [unwired: 2 out]
            n112 = local read "Output Amp #1"() -> (w348:dbl)
            n113 = Not Equal?(x=w348, y=w349) -> (x != y?=w354:bool)
            n114 = And(x=w350, y=w354) -> (x .and. y?=w355:bool)
            n115 = case shown="True" w355 {
              tunnel: w353 -> [w357 w368]
              tunnel: [w357 w367] -> w352
              tunnel: w348 -> [_ w359]
              tunnel: w347 -> [w356 w360]
              tunnel: [w356 w358] -> w346
              frame False {
              }
              frame True {
                n116 = local read "SR830 #1 Manual \nPhase"() -> (w366:dbl)
                n117 = local read "SR830 #1 \nAuto Phase"() -> (w365:bool)
                n118 = local read "SR830 #1 Detection Harm. Num."() -> (w363:dbl)
                n119 = local read "External Reference Trigger (0: Sine Zero Crossing)"() -> (w361:u16)
                n120 = local read "SR830 #1 Reference Source"() -> (w364:u16)
                n121 = local read "SR830 #1 Internal \nReference Frequency"() -> (w362:dbl)
                n122 = Unbundle(w368) -> ("Reference & Errors"=w370:T2)  [unwired: 2 out]
                n123 = Unbundle(w370) -> ("VISA resource name out"=w374:refnum<visa-resource-name>, "error out"=w373:errorcluster)
                n124 = Bundle(cluster=w360, "Voltage Output"=w359) -> (w358:T5)  [unwired: 2 in]
                n125 = call <instrlib>:"Configure Reference.vi"("VISA resource name"=w374, "Auto Phase (T: Enabled)"=w365, "Manual Phase (0 Degree)"=w366, "Reference Source (1: Internal)"=w364, "Sine Output Amplitude (1 V)"=w359, "Detection Harmonic Number (1)"=w363, "error in (no error)"=w373, "Internal Reference Frequency (1000 Hz)"=w362, "External Reference Trigger (0: Sine Zero Crossing)"=w361) -> ("VISA resource name out"=w372:refnum<visa-resource-name>, "error out"=w371:errorcluster)  [unwired: 5 in]
                n126 = Bundle(cluster=w370, "VISA resource name out"=w372, "error out"=w371) -> (w369:T2)
                n127 = Bundle(cluster=w368, "Reference & Errors"=w369) -> (w367:T4)  [unwired: 2 in]
              }
            }
          }
          frame #1 {
            n128 = Unbundle(w381) -> ("Initialised?"=w380:bool)  [unwired: 2 out]
            n129 = Unbundle(w376) -> ("Voltage Output"=w379:dbl)  [unwired: 2 out]
            n130 = local read "Output Amp #2"() -> (w377:dbl)
            n131 = Not Equal?(x=w377, y=w379) -> (x != y?=w383:bool)
            n132 = And(x=w380, y=w383) -> (x .and. y?=w384:bool)
            n133 = case shown="True" w384 {
              tunnel: w382 -> [w386 w396]
              tunnel: [w386 w397] -> w378
              tunnel: w377 -> [_ w388]
              tunnel: w376 -> [w385 w389]
              tunnel: [w385 w387] -> w375
              frame False {
              }
              frame True {
                n134 = local read "SR830 #2 Internal \nReference Frequency"() -> (w395:dbl)
                n135 = local read "External Reference Trigger #2 (0: Sine Zero Crossing)"() -> (w394:u16)
                n136 = local read "SR830 #2 Detection Harm. Num."() -> (w393:dbl)
                n137 = local read "SR830 #2 Reference Source"() -> (w392:u16)
                n138 = local read "SR830 #2 \nAuto Phase"() -> (w391:bool)
                n139 = local read "SR830 #2 Manual \nPhase"() -> (w390:dbl)
                n140 = Unbundle(w396) -> ("Reference & Errors"=w399:T2)  [unwired: 2 out]
                n141 = Unbundle(w399) -> ("VISA resource name out"=w403:refnum<visa-resource-name>, "error out"=w402:errorcluster)
                n142 = Bundle(cluster=w389, "Voltage Output"=w388) -> (w387:T5)  [unwired: 2 in]
                n143 = call <instrlib>:"Configure Reference.vi"("VISA resource name"=w403, "Auto Phase (T: Enabled)"=w391, "Manual Phase (0 Degree)"=w390, "Reference Source (1: Internal)"=w392, "Sine Output Amplitude (1 V)"=w388, "Detection Harmonic Number (1)"=w393, "error in (no error)"=w402, "Internal Reference Frequency (1000 Hz)"=w395, "External Reference Trigger (0: Sine Zero Crossing)"=w394) -> ("VISA resource name out"=w401:refnum<visa-resource-name>, "error out"=w400:errorcluster)  [unwired: 5 in]
                n144 = Bundle(cluster=w399, "VISA resource name out"=w401, "error out"=w400) -> (w398:T2)
                n145 = Bundle(cluster=w396, "Reference & Errors"=w398) -> (w397:T4)  [unwired: 2 in]
              }
            }
          }
          frame #2 {
            n146 = Unbundle(w411) -> ("Initialised?"=w410:bool)  [unwired: 2 out]
            n147 = Unbundle(w405) -> ("Voltage Output"=w409:dbl)  [unwired: 2 out]
            n148 = local read "Output Amp #3"() -> (w406:dbl)
            n149 = Not Equal?(x=w406, y=w409) -> (x != y?=w412:bool)
            n150 = And(x=w410, y=w412) -> (x .and. y?=w413:bool)
            n151 = case shown="False" w413 {
              tunnel: w408 -> [w415 w426]
              tunnel: [w415 w425] -> w407
              tunnel: w406 -> [_ w417]
              tunnel: w405 -> [w414 w418]
              tunnel: [w414 w416] -> w404
              frame False {
              }
              frame True {
                n152 = local read "SR830 #3 Manual \nPhase"() -> (w421:dbl)
                n153 = local read "SR830 #3 \nAuto Phase"() -> (w422:bool)
                n154 = local read "SR830 #3 Internal \nReference Frequency"() -> (w419:dbl)
                n155 = local read "SR830 #3 Detection Harm. Num."() -> (w420:dbl)
                n156 = local read "External Reference Trigger (0: Sine Zero Crossing)  2"() -> (w424:u16)
                n157 = local read "SR830 #3 Reference Source"() -> (w423:u16)
                n158 = Unbundle(w426) -> ("Reference & Errors"=w428:T2)  [unwired: 2 out]
                n159 = Bundle(cluster=w418, "Voltage Output"=w417) -> (w416:T5)  [unwired: 2 in]
                n160 = Unbundle(w428) -> ("VISA resource name out"=w432:refnum<visa-resource-name>, "error out"=w431:errorcluster)
                n161 = call <instrlib>:"Configure Reference.vi"("VISA resource name"=w432, "Auto Phase (T: Enabled)"=w422, "Manual Phase (0 Degree)"=w421, "Reference Source (1: Internal)"=w423, "Sine Output Amplitude (1 V)"=w417, "Detection Harmonic Number (1)"=w420, "error in (no error)"=w431, "Internal Reference Frequency (1000 Hz)"=w419, "External Reference Trigger (0: Sine Zero Crossing)"=w424) -> ("VISA resource name out"=w430:refnum<visa-resource-name>, "error out"=w429:errorcluster)  [unwired: 5 in]
                n162 = Bundle(cluster=w428, "VISA resource name out"=w430, "error out"=w429) -> (w427:T2)
                n163 = Bundle(cluster=w426, "Reference & Errors"=w427) -> (w425:T4)  [unwired: 2 in]
              }
            }
          }
        }
      }
      frame #3 {
        # "Auto change sensitivity"
        n164 = stacked-sequence {
          seq-local: [_ w502 _] -> [_ _ w562]
          seq-local: [w447 _ _] -> [_ w501 _]
          seq-local: [w446 _ _] -> [_ w506 _]
          seq-local: [_ w503 _] -> [_ _ w557]
          tunnel: w444 -> [w450 _ _]
          tunnel: [_ _ w558] -> w443
          tunnel: [_ _ w561] -> w442
          tunnel: w441 -> [w449 w505 w560]
          tunnel: w434 -> [w445 _ _]
          frame #0 {
            n165 = Unbundle(w449) -> ("Initialised?"=w448:bool)  [unwired: 2 out]
            n166 = case shown="True" w448 {
              tunnel: w450 -> [w452 w461]
              tunnel: [w452 w460] -> w447
              tunnel: [w451 w457] -> w446
              tunnel: w445 -> [w451 w454]
              frame False {
              }
              frame True {
                n167 = Unbundle(w461) -> ("Sensitivity"=w464:i16)  [unwired: 2 out]
                n168 = call "SR830_sensitivity_de-enumerator.vi"("Sensitivity (Initial Value)"=w464) -> ("Sensitivity (nV/fA)"=w462:dbl)  [unwired: 10 in]
                n169 = local read "R-Value"() -> (w453:dbl)
                n170 = Divide(x=w462, y=1000000000.0) -> (x/y=w465:dbl)
                n171 = Absolute Value(x=w453) -> (abs(x)=w455:dbl)
                n172 = Multiply(x=w465, y=0.9) -> (x*y=w473:dbl)
                n173 = Multiply(x=w465, y=0.25) -> (x*y=w472:dbl)
                n174 = Less?(x=w455, y=w472) -> (x < y?=w469:bool)
                "Sense Under" <- w469
                n175 = Greater?(x=w455, y=w473) -> (0:w468:bool)
                "Sense Over" <- w468
                n176 = Or(x=w469, y=w468) -> (x .or. y?=w467:bool)
                n177 = case shown="True" w469 {
                  tunnel: w464 -> [w497 w500]
                  tunnel: [w497 w498] -> w471
                  frame False {
                  }
                  frame True {
                    n178 = Subtract(x=w500, y=i16 1) -> (x-y=w498:i16)
                  }
                }
                n179 = local read "SR830 #1 \nDynamic Reserve"() -> (w463:i16)
                n180 = case shown="True" w468 {
                  tunnel: w471 -> [w493 w496]
                  tunnel: [w493 w494] -> w470
                  frame False {
                  }
                  frame True {
                    n181 = Add(x=w496, y=i16 1) -> (x+y=w494:i16)
                  }
                }
                n182 = Unbundle(w454) -> ("Reference & Errors"=w459:T2)  [unwired: 2 out]
                n183 = case shown="True" w467 {
                  tunnel: w470 -> [w477 w485]
                  tunnel: [w477 w485] -> w456
                  tunnel: w463 -> [_ w492]
                  tunnel: w459 -> [w476 w480]
                  tunnel: [w476 w488] -> w458
                  frame False {
                  }
                  frame True {
                    n184 = local read "SR830 #1 \nTime Constant"() -> (w484:u16)
                    n185 = call "SR830_time_constant_de-enumerator.vi"("Time Constant (8: 100ms)"=w484) -> ("Time Constant (us)"=w483:dbl)  [unwired: 10 in]
                    n186 = Divide(x=w483, y=1000000.0) -> (x/y=w481:dbl)
                    n187 = Unbundle(w480) -> ("VISA resource name out"=w479:refnum<visa-resource-name>, "error out"=w478:errorcluster)
                    n188 = call <instrlib>:"Configure Sensitivity and Reserve.vi"("error in (no error)"=w478, "Sensitivity (-1: Auto gain)"=w485, "Dynamic Reserve (-1: Auto Reserve)"=w492, "VISA resource name"=w479) -> ("error out"=w487:errorcluster, "VISA resource name out"=w489:refnum<visa-resource-name>)  [unwired: 6 in]
                    n189 = Multiply(x=w481, y=3.0) -> (x*y=w491:dbl)
                    n190 = call "Time Delay"("error in (no error)"=w487, "Delay Time (s)"=w491) -> ("error out"=w486:errorcluster)  [unwired: 9 in]
                    n191 = Bundle("VISA resource name out"=w489, "error out"=w486) -> (w488:T2)  [unwired: 1 in]
                  }
                }
                n192 = Bundle(cluster=w461, "Sensitivity"=w456) -> (w460:T6)  [unwired: 2 in]
                n193 = Bundle(cluster=w454, "Reference & Errors"=w458) -> (w457:T4)  [unwired: 2 in]
              }
            }
          }
          frame #1 {
            n194 = Unbundle(w505) -> ("Initialised?"=w504:bool)  [unwired: 2 out]
            n195 = case shown="True" w504 {
              tunnel: w501 -> [w507 w520]
              tunnel: [w507 w519] -> w502
              tunnel: w506 -> [w508 w517]
              tunnel: [w508 w516] -> w503
              frame False {
              }
              frame True {
                n196 = Unbundle(w520) -> ("Sensitivity"=w512:i16)  [unwired: 2 out]
                n197 = local read "R-Value 2"() -> (w509:dbl)
                n198 = call "SR830_sensitivity_de-enumerator.vi"("Sensitivity (Initial Value)"=w512) -> ("Sensitivity (nV/fA)"=w515:dbl)  [unwired: 10 in]
                n199 = Divide(x=w515, y=1000000000.0) -> (x/y=w521:dbl)
                n200 = Absolute Value(x=w509) -> (abs(x)=w511:dbl)
                n201 = Multiply(x=w521, y=0.9) -> (x*y=w529:dbl)
                n202 = Multiply(x=w521, y=0.25) -> (x*y=w528:dbl)
                n203 = Less?(x=w511, y=w528) -> (x < y?=w525:bool)
                "Sense\nUnder 2" <- w525
                n204 = Greater?(x=w511, y=w529) -> (0:w524:bool)
                "Sense\nOver 2" <- w524
                n205 = case shown="True" w525 {
                  tunnel: [w553 w555] -> w527
                  tunnel: w512 -> [w553 w554]
                  frame False {
                  }
                  frame True {
                    n206 = Subtract(x=w554, y=i16 1) -> (x-y=w555:i16)
                  }
                }
                n207 = Or(x=w525, y=w524) -> (x .or. y?=w523:bool)
                n208 = Unbundle(w517) -> ("Reference & Errors"=w518:T2)  [unwired: 2 out]
                n209 = local read "SR830 #2 \nDynamic Reserve"() -> (w514:i16)
                n210 = case shown="True" w524 {
                  tunnel: w527 -> [w549 w552]
                  tunnel: [w549 w550] -> w526
                  frame False {
                  }
                  frame True {
                    n211 = Add(x=w552, y=i16 1) -> (x+y=w550:i16)
                  }
                }
                n212 = case shown="True" w523 {
                  tunnel: w526 -> [w533 w548]
                  tunnel: [w533 w548] -> w513
                  tunnel: w518 -> [w532 w536]
                  tunnel: [w532 w543] -> w510
                  tunnel: w514 -> [_ w541]
                  frame False {
                  }
                  frame True {
                    n213 = local read "SR830 #2 \nTime Constant"() -> (w538:u16)
                    n214 = call "SR830_time_constant_de-enumerator.vi"("Time Constant (8: 100ms)"=w538) -> ("Time Constant (us)"=w540:dbl)  [unwired: 10 in]
                    n215 = Unbundle(w536) -> ("VISA resource name out"=w535:refnum<visa-resource-name>, "error out"=w534:errorcluster)
                    n216 = Divide(x=w540, y=1000000.0) -> (x/y=w537:dbl)
                    n217 = call <instrlib>:"Configure Sensitivity and Reserve.vi"("error in (no error)"=w534, "Sensitivity (-1: Auto gain)"=w548, "Dynamic Reserve (-1: Auto Reserve)"=w541, "VISA resource name"=w535) -> ("error out"=w544:errorcluster, "VISA resource name out"=w545:refnum<visa-resource-name>)  [unwired: 6 in]
                    n218 = Multiply(x=w537, y=3.0) -> (x*y=w547:dbl)
                    n219 = call "Time Delay2"("error in (no error)"=w544, "Delay Time (s)"=w547) -> ("error out"=w542:errorcluster)  [unwired: 9 in]
                    n220 = Bundle("VISA resource name out"=w545, "error out"=w542) -> (w543:T2)  [unwired: 1 in]
                  }
                }
                n221 = Bundle(cluster=w520, "Sensitivity"=w513) -> (w519:T6)  [unwired: 2 in]
                n222 = Bundle(cluster=w517, "Reference & Errors"=w510) -> (w516:T4)  [unwired: 2 in]
              }
            }
          }
          frame #2 {
            n223 = Unbundle(w560) -> ("Initialised?"=w559:bool)  [unwired: 2 out]
            n224 = case shown="True" w559 {
              tunnel: w562 -> [w564 w569]
              tunnel: [w564 w575] -> w558
              tunnel: [w563 w573] -> w561
              tunnel: w557 -> [w563 w568]
              frame False {
              }
              frame True {
                n225 = Unbundle(w569) -> ("Sensitivity"=w567:i16)  [unwired: 2 out]
                n226 = local read "R-Value 3"() -> (w565:dbl)
                n227 = Unbundle(w568) -> ("Reference & Errors"=w574:T2)  [unwired: 2 out]
                n228 = call "SR830_sensitivity_de-enumerator.vi"("Sensitivity (Initial Value)"=w567) -> ("Sensitivity (nV/fA)"=w571:dbl)  [unwired: 10 in]
                n229 = Divide(x=w571, y=1000000000.0) -> (x/y=w576:dbl)
                n230 = Absolute Value(x=w565) -> (abs(x)=w566:dbl)
                n231 = Multiply(x=w576, y=0.9) -> (x*y=w584:dbl)
                n232 = Multiply(x=w576, y=0.25) -> (x*y=w583:dbl)
                n233 = Less?(x=w566, y=w583) -> (x < y?=w580:bool)
                "Sense\nUnder 3" <- w580
                n234 = Greater?(x=w566, y=w584) -> (0:w579:bool)
                "Sense\nOver 3" <- w579
                n235 = case shown="True" w580 {
                  tunnel: [w608 w610] -> w582
                  tunnel: w567 -> [w608 w609]
                  frame False {
                  }
                  frame True {
                    n236 = Subtract(x=w609, y=i16 1) -> (x-y=w610:i16)
                  }
                }
                n237 = Or(x=w580, y=w579) -> (x .or. y?=w578:bool)
                n238 = local read "SR830 #3 \nDynamic Reserve"() -> (w572:i16)
                n239 = case shown="True" w579 {
                  tunnel: w582 -> [w604 w607]
                  tunnel: [w604 w605] -> w581
                  frame False {
                  }
                  frame True {
                    n240 = Add(x=w607, y=i16 1) -> (x+y=w605:i16)
                  }
                }
                n241 = case shown="True" w578 {
                  tunnel: w581 -> [w588 w603]
                  tunnel: [w588 w603] -> w570
                  tunnel: w574 -> [w587 w591]
                  tunnel: [w587 w597] -> _
                  tunnel: w572 -> [_ w596]
                  frame False {
                  }
                  frame True {
                    n242 = local read "SR830 #3 \nTime Constant"() -> (w593:u16)
                    n243 = call "SR830_time_constant_de-enumerator.vi"("Time Constant (8: 100ms)"=w593) -> ("Time Constant (us)"=w595:dbl)  [unwired: 10 in]
                    n244 = Unbundle(w591) -> ("VISA resource name out"=w590:refnum<visa-resource-name>, "error out"=w589:errorcluster)
                    n245 = Divide(x=w595, y=1000000.0) -> (x/y=w592:dbl)
                    n246 = call <instrlib>:"Configure Sensitivity and Reserve.vi"("error in (no error)"=w589, "Sensitivity (-1: Auto gain)"=w603, "Dynamic Reserve (-1: Auto Reserve)"=w596, "VISA resource name"=w590) -> ("error out"=w602:errorcluster, "VISA resource name out"=w598:refnum<visa-resource-name>)  [unwired: 6 in]
                    n247 = Multiply(x=w592, y=3.0) -> (x*y=w601:dbl)
                    n248 = call "Time Delay3"("error in (no error)"=w602, "Delay Time (s)"=w601) -> ("error out"=w599:errorcluster)  [unwired: 9 in]
                    n249 = Bundle("VISA resource name out"=w598, "error out"=w599) -> (w597:T2)  [unwired: 1 in]
                  }
                }
                n250 = Bundle(cluster=w569, "Sensitivity"=w570) -> (w575:T6)  [unwired: 2 in]
                n251 = Bundle(cluster=w568) -> (w573:T4)  [unwired: 3 in]
              }
            }
          }
        }
        n252 = Unbundle(w443) -> ("Sensitivity"=w439:i16, "Sensitivity"=w438:i16, "Sensitivity"=w436:i16)
        n253 = call "SR830_sensitivity_de-enumerator.vi"("Sensitivity (Initial Value)"=w439) -> ("Sensitivity (nV/fA)"=→"SR830 #3 Sensitivity":dbl)  [unwired: 10 in]
        n254 = call "SR830_sensitivity_de-enumerator.vi"("Sensitivity (Initial Value)"=w436) -> ("Sensitivity (nV/fA)"=→"SR830 #3 Sensitivity 3":dbl)  [unwired: 10 in]
        n255 = call "SR830_sensitivity_de-enumerator.vi"("Sensitivity (Initial Value)"=w438) -> ("Sensitivity (nV/fA)"=→"SR830 #3 Sensitivity 2":dbl)  [unwired: 10 in]
      }
    }
    n256 = Wait (ms)(milliseconds to wait="Loop Timing (ms)") -> ()  [unwired: 1 out]
    "Device Intialization" <- w38
  }
  n257 = local write "program_stop"(FALSE ("program_stop")) -> ()
  n258 = Unbundle(w11) -> ("Reference & Errors"=w7:T2, "Reference & Errors"=w6:T2, "Reference & Errors"=w5:T2)
  n259 = Unbundle(w12) -> ("Initialised?"=w10:bool, "Initialised?"=w9:bool, "Initialised?"=w8:bool)
  n260 = case shown="True" w10 {
    tunnel: w7 -> [_ w612]
    frame False {
    }
    frame True {
      n261 = Unbundle(w612) -> ("VISA resource name out"=w614:refnum<visa-resource-name>, "error out"=w613:errorcluster)
      n262 = call <instrlib>:"Close.vi"("error in (no error)"=w613, "VISA resource name"=w614) -> ("error out"=w615:errorcluster)  [unwired: 9 in]
      n263 = call <vilib>:"Simple Error Handler.vi"("error in (no error)"=w615) -> ()  [unwired: 4 in, 5 out]
    }
  }
  n264 = case shown="True" w9 {
    tunnel: w6 -> [_ w616]
    frame False {
    }
    frame True {
      n265 = Unbundle(w616) -> ("VISA resource name out"=w618:refnum<visa-resource-name>, "error out"=w617:errorcluster)
      n266 = call <instrlib>:"Close.vi"("error in (no error)"=w617, "VISA resource name"=w618) -> ("error out"=w619:errorcluster)  [unwired: 9 in]
      n267 = call <vilib>:"Simple Error Handler.vi"("error in (no error)"=w619) -> ()  [unwired: 4 in, 5 out]
    }
  }
  n268 = case shown="True" w8 {
    tunnel: w5 -> [_ w620]
    frame False {
    }
    frame True {
      n269 = Unbundle(w620) -> ("VISA resource name out"=w622:refnum<visa-resource-name>, "error out"=w621:errorcluster)
      n270 = call <instrlib>:"Close.vi"("error in (no error)"=w621, "VISA resource name"=w622) -> ("error out"=w623:errorcluster)  [unwired: 9 in]
      n271 = call <vilib>:"Simple Error Handler.vi"("error in (no error)"=w623) -> ()  [unwired: 4 in, 5 out]
    }
  }
